vi "_PC_RTFunc_AccessExtAO.vi"(7 "Function":enum16{"Init", "Write", "Read"}(ring)=enum."Write", 8 "error in (no error)":errorcluster, 10 "AnalogueOutput in":T1=[{"Label"="", "y"=0.0}, {"Label"="", "y"=0.0}, {"Label"="", "y"=0.0}, {"Label"="", "y"=0.0}, {"Label"="", "y"=0.0}, {"Label"="", "y"=0.0}, {"Label"="", "y"=0.0}, {"Label"="", "y"=0.0}]) -> (0 "error out":errorcluster, 2 "AnalogueOutput out":T1)   [LabVIEW 2018]
uses:
  RT/PublicSubVI/Ctl/_ctl_RT_ExtAO.ctl
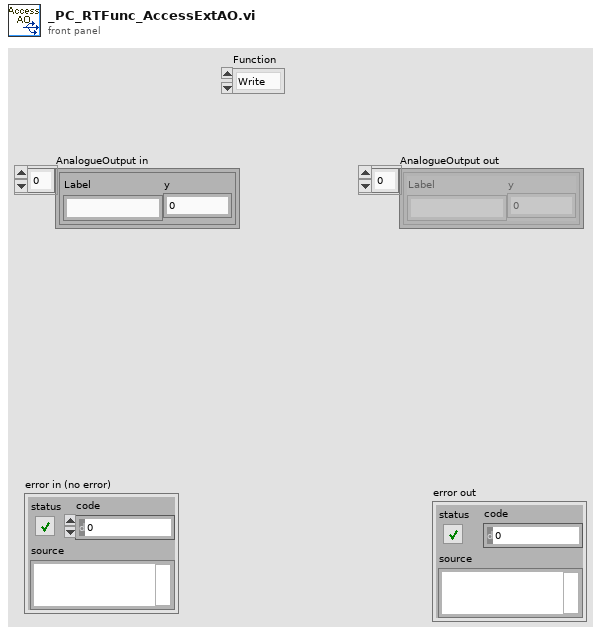
[diagram p1: front panel]
types:
  T1 = typedef "_ctl_RT_ExtAO.ctl" = cluster{"Label":string, "y":dbl}[]
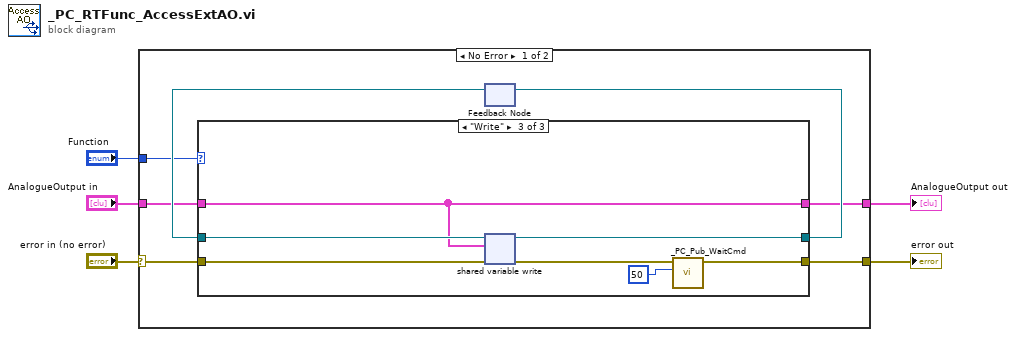
[diagram p0: block diagram]
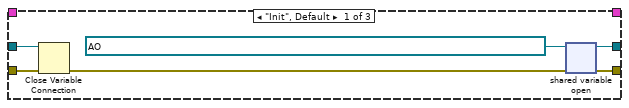
[diagram p2: hidden frame]
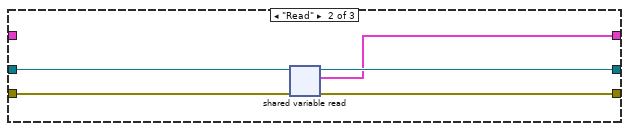
[diagram p3: hidden frame]
diagram:
  n1 = case shown="No Error" "error in (no error)" {
    selector: "error in (no error)" -> [w9 w31]
    tunnel: [w12 w31] -> w5
    tunnel: "Function" -> [w8 _]
    tunnel: [w7 _] -> w2
    tunnel: "AnalogueOutput in" -> [w6 _]
    frame No Error {
      n2 = feedback #1() -> (w10:refnum<k21>)  [unwired: 1 in]
      n3 = case shown="\"Write\"" w8 {
        tunnel: w10 -> [w15 w23 w30]
        tunnel: w9 -> [w14 w22 w29]
        tunnel: [w18 w21 w28] -> w11
        tunnel: [w17 w19 w24] -> w12
        tunnel: [_ w20 w27] -> w7
        tunnel: w6 -> [_ _ w27]
        frame "Init", Default {
          n4 = Close Variable Connection(8:w14, 11:w15) -> (0:w13:errorcluster)
          n5 = shared-variable-open(refnum<k21> "ni.var.psp://NI-sbRIO/_RT_CtrlLoop_DigitalAnalogueOutput_Variables/ExtAO" ("shared variable refnum in"), w13) -> (w18:refnum<k21>, w17:errorcluster)
        }
        frame "Read" {
          n6 = shared-variable-read(w23, w22) -> (w21:refnum<k21>, w19:errorcluster, w20:T1)  [unwired: 1 out]
        }
        frame "Write" {
          n7 = shared-variable-write(w30, w29, w27) -> (w28:refnum<k21>, w25:errorcluster)
          n8 = call "_PC_Pub_WaitCmd.vi"("milliseconds to wait"=u32 50, "error in (no error)"=w25) -> ("error out"=w24:errorcluster)  [unwired: 9 in]
        }
      }
      n9 = feedback-in #1(w11) -> ()
    }
    frame Error {
    }
  }
  "error out" <- w5
  "AnalogueOutput out" <- w2
